vi "querey source settings menu.vi"(0 "Enable":bool=TRUE, 1 "subvi?":bool, 5 "error in (no error)":errorcluster) -> (14 "Output cluster":T2={"Integer Timestamp"=0, "Einzel Voltage"=0.0, "Needle Voltage"=0.0, "Frequency"=1.0, "Width (ms) : 0.1 "=0.05, "Desired Amplitude (V)"=0.0, "X Voltage"=0.0, "Y Voltage"=0.0, "Settings ID"="", "ID#"=0} {"Needle Voltage" min=0.0 max=10.0 step=0.01 format="%.2g"; "Y Voltage" min=0.0 max=9.0 step=0.01 format="%.2g"; "X Voltage" min=0.0 max=9.0 step=0.01 format="%.2g"; "Einzel Voltage" min=0.0 max=10.0 step=0.01 format="%.2g"; "Desired Amplitude (V)" min=0.0 max=10.0 step=0.01 format="%5.2f"; "Width (ms) : 0.1" min=0.05 max=5.0 step=0.01 format="%6.2f"; "Frequency" min=1.0 max=100.0 step=0.01 format="%.1f"}, 15 "Cancel loading":bool caption="Cancel", 18 "OK":bool, 19 "error out":errorcluster)   [LabVIEW 2012]
doc: "Displays a standard dialog box that prompts users to enter information, such as a user name and password.\n--------------------\n\nThis Express VI is configured as follows:\n\nMessage to Display to the User:\nThe inputs are: \nNumber: Upper Timestamp Range\nNumber: Lower Timestamp Range\nNumber: Settings ID"
uses:
  dust_soruce_control.ctl
  <vilib>/addons/database/Auxilliary.llb/DB Tools Cursor Type.ctl
  <vilib>/addons/database/Connection.llb/Conn Execute.vi
  <vilib>/addons/database/Recordset.llb/Rec Fetch Recordset Data (R).vi
  <vilib>/addons/database/Recordset.llb/Rec Destroy - Connection.vi
  <vilib>/addons/database/_DB Variant To Data/Database Variant To Data.xnode
  <vilib>/addons/database/NI_Database_API.lvlib
panel:
  in  "Clear Filter":bool
  in  "Tag Filter":T1
  in  "Settings ID Type":enum32{"All", "Saved", "Automatic"}(radio)
  in  "OK2":bool
  in  "Cancel":bool
  in  "Settings ID":i32(ring) items=["Any Settings ID."=-1, "Automatic Update (DT: Graphite-2-1; HV: 0.0; Time: 2/13/2014 10:09:24 AM)"=114, "Automatic Update (DT: Graphite-2-1; HV: 0.0; Time: 2/13/2014 10:09:22 AM)"=113, "Automatic Update (DT: Graphite-2-1; HV: 0.0; Time: 2/13/2014 10:09:19 AM)"=112, "Automatic Update (DT: Graphite-2-1; HV: 0.0; Time: 2/13/2014 9:57:29 AM)"=111, "Automatic Update (DT: Graphite-2-1; HV: 0.0; Time: 2/13/2014 9:57:27 AM)"=110, "Automatic Update (DT: Graphite-2-1; HV: 0.0; Time: 2/12/2014 2:14:33 PM)"=109, "Automatic Update (DT: Graphite-2-1; HV: 0.0; Time: 2/12/2014 2:14:18 PM)"=108, "Automatic Update (DT: Graphite-2-1; HV: 0.0; Time: 2/12/2014 1:53:33 PM)"=107, "Automatic Update (DT: DT: Graphite-2-1; HV: 0.0; Time: 2/12/2014 1:52:08 PM)"=106, "Automatic Update at  10/25/2012 3:24:21 PM"=100, "Automatic Update at  10/25/2012 3:14:43 PM"=99, "Automatic Update at  10/24/2012 5:17:54 PM"=98, "Automatic Update at  10/24/2012 5:05:57 PM"=96, "Automatic Update at  10/24/2012 4:27:19 PM"=95, "Automatic Update at  10/24/2012 4:13:56 PM"=94, "Automatic Update at  10/24/2012 3:47:44 PM"=90]
  in  "Lower Timestamp Range":timestamp
  in  "Upper Timestamp Range":timestamp
  out "Settings":cluster{"String":string, "Value":dbl}[](array[cluster])
  in  "Einzel Voltage":dbl
  in  "Needle Voltage":dbl
  in  "Frequency":dbl
  in  "Width (ms) : 0.1":dbl
  in  "Desired Amplitude (V)":dbl
  in  "X Voltage":dbl
  in  "Y Voltage":dbl
  out "Settings to be loaded":string
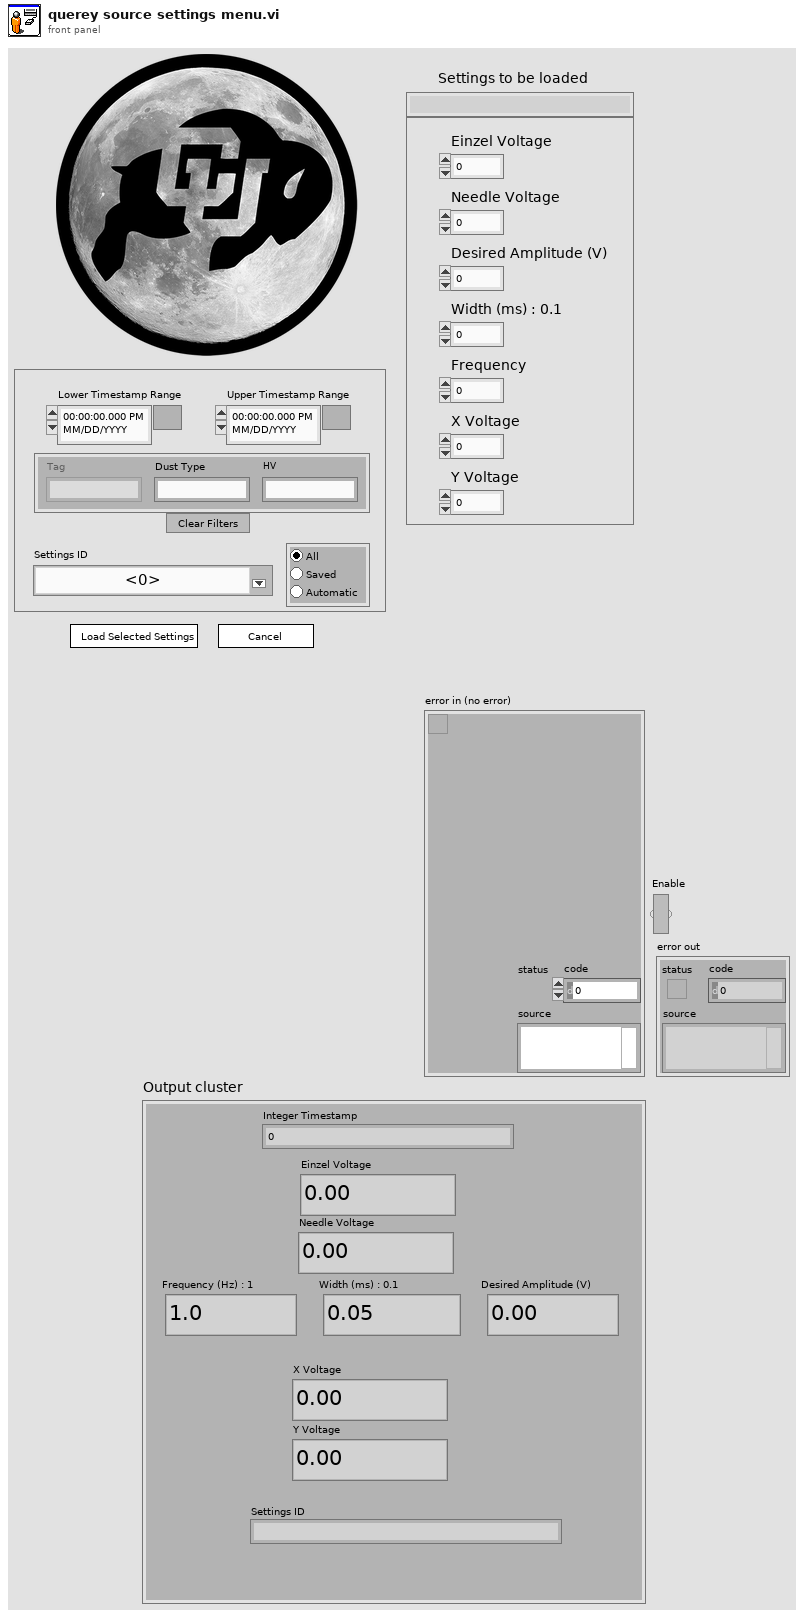
[diagram p1: front panel]
types:
  T1 = cluster{"Tag":string, "Dust Type":string, "HV":string}
  T2 = typedef "dust_soruce_control.ctl" = cluster{"Integer Timestamp":u64, "Einzel Voltage":dbl, "Needle Voltage":dbl, "Frequency":dbl, "Width (ms) : 0.1 ":dbl, "Desired Amplitude (V)":dbl, "X Voltage":dbl, "Y Voltage":dbl, "Settings ID":string, "ID#":i32}
  T3 = enum32{"Invalid", "Standard", "Closed", "Hidden", "Minimized", "Maximized"}
  T4 = enum8{"Enabled", "Disabled", "Disabled and Grayed Out"}
  T5 = typedef "NI_Database_API.lvlib/DB Tools Cursor Type.ctl" = enum16{"forward-only", "keyset", "dynamic", "static"}
  T6 = typedef "NI_Database_API.lvlib/Conn ObjectReference.ctl" = refnum<k1>
  T7 = typedef "NI_Database_API.lvlib/Rec ObjectReference.ctl" = refnum<k1>
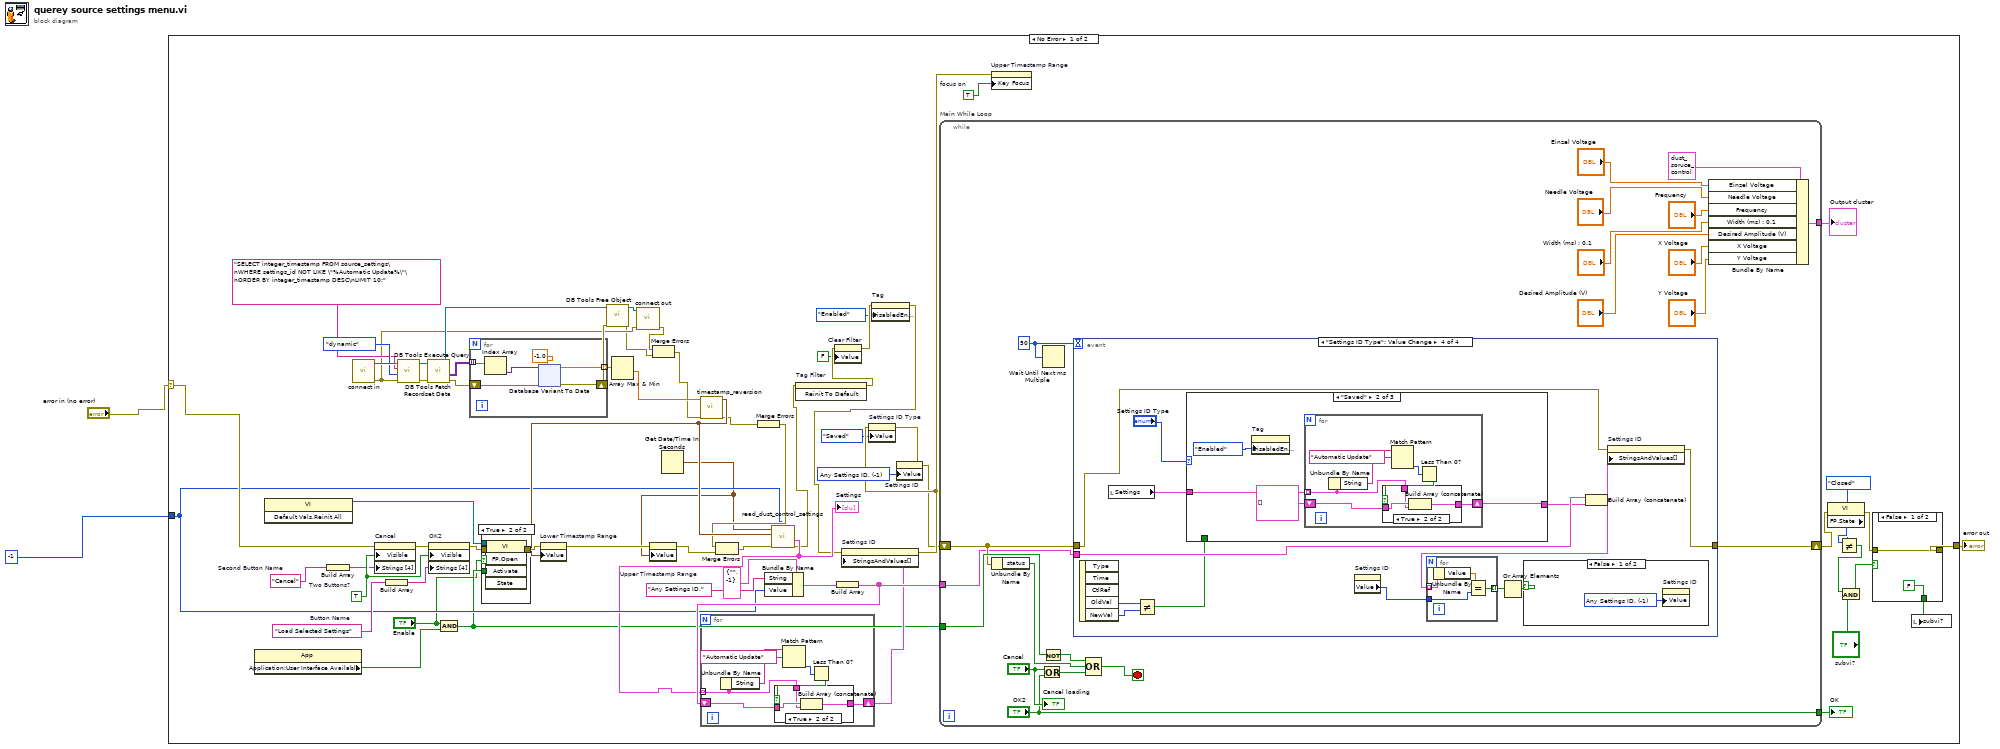
[diagram p0: block diagram]
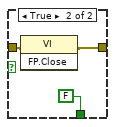
[diagram p3: hidden frame]
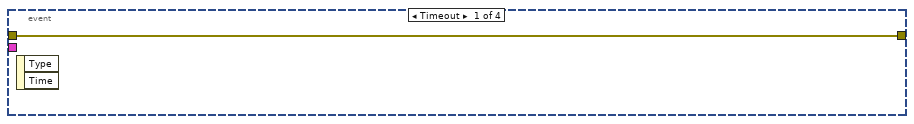
[diagram p5: hidden frame]
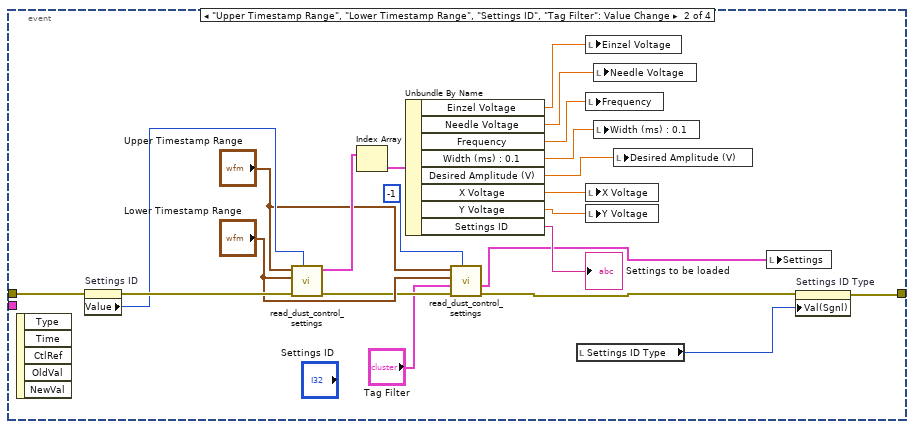
[diagram p6: hidden frame]
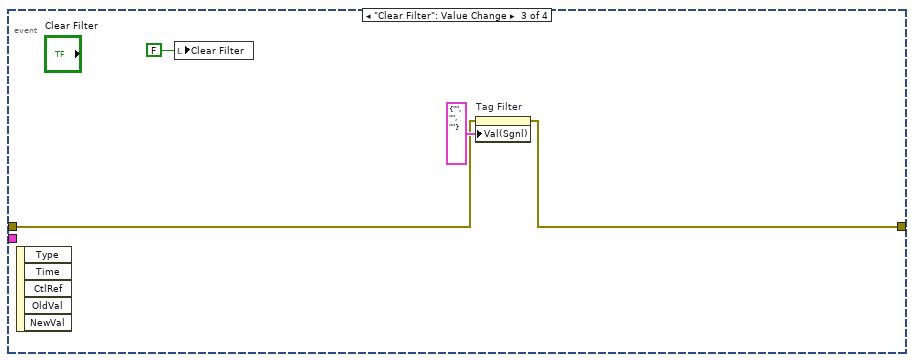
[diagram p7: hidden frame]
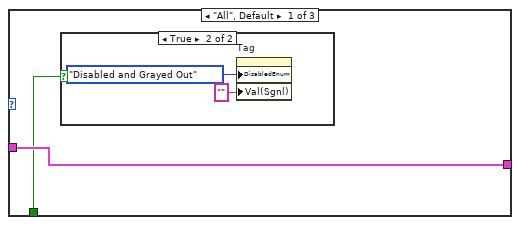
[diagram p9: hidden frame]
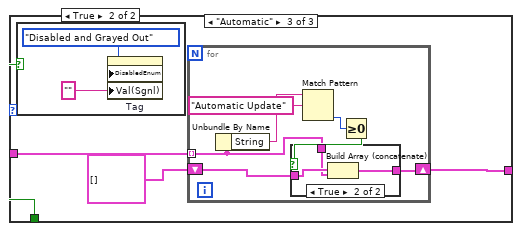
[diagram p12: hidden frame]
diagram:
  n1 = case shown="No Error" "error in (no error)" {
    selector: "error in (no error)" -> [w53 w230]
    tunnel: [w28 w230] -> w3
    tunnel: -1 ("Settings to be loaded") -> [w27 _]
    frame No Error {
      w22 = -1 items=["Any Settings ID."=-1, "Anna's Settings"=86, "Anna's Settings1"=87, "Test 'Test' \"Test\" test test."=97, "Test\""=91, "Test\""=92, "test 3"=82, "test 4"=83, "test mctesty"=88, "test mctesty"=89, "this is a \"test\" setting"=93] ("Settings ID")
      w61 = TRUE  # focus on
      w65 = "Cancel"  # Second Button Name
      w63 = "Load Selected Settings"  # Button Name
      w69 = TRUE  # Two Buttons?
      n2 = property class="App"() -> ("Application:User Interface Available"=w62:bool)  [unwired: 2 in, 2 out]
      n3 = invoke class="VI" method="Default Vals.Reinit All"() -> (reference out=w9:refnum<vi>)  [unwired: 3 in, 2 out]
      n4 = Build Array(w65) -> (w66:string[])
      n5 = call "connect in.vi"() -> ("error out"=w38:errorcluster, "Database Connection"=w48:T6)  [unwired: 7 in, 1 out]
      n6 = property on="Cancel" class="Bool"(error in=w53, "Visible"=w69, "Strings [4]"=w66) -> (error out=w67:errorcluster)  [unwired: 1 in, 1 out]
      n7 = Build Array(w63) -> (w64:string[])
      n8 = call-poly <vilib>:"DB Tools Execute Query.vi"("error in (no error)"=w38, "cursor type"=DB_Tools_Cursor_Type."dynamic", "SQL query"="SELECT integer_timestamp FROM source_settings\nWHERE settings_id NOT LIKE \"%Automatic Update%\"\nORDER BY integer_timestamp DESC\nLIMIT 10;" ("string"), "connection reference"=w48) -> ("error out"=w49:errorcluster, "recordset reference"=w50:T7)  [unwired: 4 in]
      n9 = call-poly <vilib>:"DB Tools Fetch Recordset Data.vi"("error in (no error)"=w49, "recordset reference"=w50) -> ("error out"=w44:errorcluster, "recordset data"=w45:variant[][], "recordset reference out"=w40:T7)  [unwired: 3 in]
      n10 = property on="OK2" class="Bool"(error in=w67, "Visible"=w69, "Strings [4]"=w64) -> (error out=w60:errorcluster)  [unwired: 1 in, 1 out]
      n11 = And(x="Enable", y=w62) -> (x .and. y?=w21:bool)
      n12 = for {
        tunnel: w45 -> [w95] mode=indexing
        tunnel: [w93] -> w43 mode=indexing
        shift-right: [w91] -> w39
        shift-left: w44 -> [w92]
        n13 = Index Array(array=w95) -> (element=w94:variant)  [unwired: 1 in]
        n14 = xnode "Database Variant To Data"("database variant"=w94, "error in (no error)"=w92, "type"=-1.0 ("Settings to be loaded")) -> ("data"=w93:dbl, "error out"=w91:errorcluster)
      }
      n15 = case shown="True" "Enable" {
        tunnel: w9 -> [_ w74]
        tunnel: w60 -> [w70 w73]
        tunnel: [w70 w72] -> w57
        tunnel: w21 -> [_ w71]
        frame False {
        }
        frame True {
          n16 = invoke class="VI" method="FP.Open"(reference=w74, error in=w73, "Activate"=w71) -> (error out=w72:errorcluster)  [unwired: 2 in, 4 out]
        }
      }
      n17 = call-poly <vilib>:"DB Tools Free Object.vi"("error in (no error)"=w39, "recordset reference"=w40) -> ("error out"=w37:errorcluster, "connection reference"=w41:T6)  [unwired: 8 in]
      n18 = Array Max & Min(array=w43) -> (min value=w42:dbl)  [unwired: 3 out]
      n19 = call "connect out.vi"("error in (no error)"=w38, "connection reference"=w41) -> ("error out"=w36:errorcluster)  [unwired: 9 in]
      n20 = Merge Errors(w36, w37) -> (w35:errorcluster)
      n21 = Get Date/Time In Seconds() -> (seconds since 1Jan1904=w18:timestamp)
      n22 = call "timestamp_reversion.vi"("error in (no error)"=w35, "Integer Timestamp"=w42) -> ("error out"=w33:errorcluster, "time stamp"=w34:timestamp)  [unwired: 7 in]
      n23 = property on="Lower Timestamp Range" class="AbsTime (strict)"(error in=w57, "Value"=w34) -> (error out=w58:errorcluster)  [unwired: 1 in, 1 out]
      n24 = property on="Upper Timestamp Range" class="AbsTime (strict)"(error in=w58, "Value"=w18) -> (error out=w32:errorcluster)  [unwired: 1 in, 1 out]
      n25 = Merge Errors(w33) -> (w31:errorcluster)
      n26 = Merge Errors(w31, w32) -> (w30:errorcluster)
      n27 = Bundle By Name(cluster=cluster{"String":string, "Value":i32} {"String"="", "Value"=-1}, "String"="Any Settings ID." ("Settings to be loaded"), "Value"=w27) -> (w54:cluster{"String":string, "Value":i32})
      n28 = call "read_dust_control_settings.vi"("Settings to be loaded"=w27, "error in (no error)"=w30, "Lower Timestamp Range"=w34, "Upper Timestamp Range"=w18) -> ("error out"=w17:errorcluster, "Array"=w25:cluster{"String":string, "Value":dbl}[])  [unwired: 5 in, 1 out]
      "Settings" <- w25
      n29 = invoke on="Tag Filter" class="Clust (strict)" method="Reinit To Default"(error in=w17) -> (error out=w16:errorcluster)  [unwired: 2 in, 2 out]
      n30 = property on="Clear Filter" class="Bool (strict)"(error in=w16, "Value"=FALSE ("Clear Filter")) -> (error out=w14:errorcluster)  [unwired: 1 in, 1 out]
      n31 = Build Array(w54) -> (w29:cluster{"String":string, "Value":i32}[])
      n32 = for {
        tunnel: w25 -> [w82] mode=indexing
        shift-right: [w81] -> w26
        shift-left: w29 -> [w83]
        n33 = Unbundle By Name(w82) -> ("String"=w86:string)
        n34 = Match Pattern(string=w86, regular expression="Automatic Update") -> (offset past match=w80:i32)  [unwired: 1 in, 3 out]
        n35 = Less Than 0?(x=w80) -> (x < 0?=w84:bool)
        n36 = case shown="True" w84 {
          tunnel: w83 -> [w87 w90]
          tunnel: w82 -> [_ w89]
          tunnel: [w87 w88] -> w81
          frame False {
          }
          frame True {
            n37 = Build Array (concatenate)(w90, w89) -> (w88:cluster{"String":string, "Value":dbl}[])
          }
        }
      }
      n38 = property on="Tag" class="Str"(error in=w14, "DisabledEnum"=T4."Enabled" ("Disabled")) -> (error out=w12:errorcluster)  [unwired: 1 in, 1 out]
      n39 = property on="Settings ID" class="Ring (strict)"(error in=w12, "StringsAndValues[]"=w26) -> (error out=w52:errorcluster)  [unwired: 1 in, 1 out]
      n40 = property on="Settings ID Type" class="RadioBtnsControl (strict)"(error in=w52, "Value"=enum32{"All", "Saved", "Automatic"}."Saved" ("Settings ID Type")) -> (error out=w24:errorcluster)  [unwired: 1 in, 1 out]
      n41 = property on="Settings ID" class="Ring (strict)"(error in=w24, "Value"=w22) -> (error out=w23:errorcluster)  [unwired: 1 in, 1 out]
      n42 = while "Main While Loop" {
        tunnel: ["OK2"] -> w68
        tunnel: w21 -> [w147]
        tunnel: w29 -> [w129]
        tunnel: [w138] -> w59
        shift-right: [w140] -> w8
        shift-left: w23 -> [w141]
        stop <- w145 stop-if-true
        w139 = u32 50 ("millisecond multiple")
        n43 = Unbundle By Name(w141) -> ("status"=w143:bool)
        n44 = Or(x="Cancel", y="OK2") -> (x .or. y?=w144:bool)
        n45 = Not(x=w147) -> (.not. x?=w146:bool)
        n46 = Wait Until Next ms Multiple(millisecond multiple=w139) -> ()  [unwired: 1 out]
        n47 = event shown="[3] \"Settings ID Type\": Value Change" {
          selector: _ -> [_ _ _ _]
          dyn-events: _ -> [_ _ _ _]
          timeout: w139 -> [_ _ _ _]
          tunnel: w141 -> [w149 w171 w173 w186]
          tunnel: [w149 w152 w172 w185] -> w140
          tunnel: w129 -> [_ _ _ w180]
          event Timeout {
            n48 = event-data() -> ()  [unwired: 1 in, 2 out]
          }
          event "Upper Timestamp Range", "Lower Timestamp Range", "Settings ID", "Tag Filter": Value Change {
            n49 = event-data() -> ()  [unwired: 1 in, 5 out]
            n50 = property on="Settings ID" class="Ring (strict)"(error in=w171) -> (error out=w170:errorcluster, "Value"=w168:i32)  [unwired: 1 in, 1 out]
            n51 = call "read_dust_control_settings.vi"("Settings to be loaded"=w168, "error in (no error)"=w170, "Lower Timestamp Range"="Lower Timestamp Range", "Upper Timestamp Range"="Upper Timestamp Range") -> ("error out"=w165:errorcluster, "Dust Source Array"=w169:T2[])  [unwired: 5 in, 1 out]
            n52 = Index Array(array=w169) -> (element=w164:T2)  [unwired: 1 in]
            n53 = Unbundle By Name(w164) -> ("Einzel Voltage"=w163:dbl, "Needle Voltage"=w162:dbl, "Frequency"=w161:dbl, "Width (ms) : 0.1"=w160:dbl, "Desired Amplitude (V)"=w159:dbl, "X Voltage"=w158:dbl, "Y Voltage"=w157:dbl, "Settings ID"=→"Settings to be loaded":string)
            n54 = call "read_dust_control_settings.vi"("Settings to be loaded"=-1, "error in (no error)"=w165, "Cluster"="Tag Filter", "Lower Timestamp Range"="Lower Timestamp Range", "Upper Timestamp Range"="Upper Timestamp Range") -> ("error out"=w153:errorcluster, "Array"=w151:cluster{"String":string, "Value":dbl}[])  [unwired: 4 in, 1 out]
            n55 = local read "Settings ID Type"() -> (w154:enum32{"All", "Saved", "Automatic"})
            n56 = local write "Einzel Voltage"(w163) -> ()
            n57 = local write "Frequency"(w161) -> ()
            n58 = local write "X Voltage"(w158) -> ()
            n59 = local write "Y Voltage"(w157) -> ()
            n60 = local write "Needle Voltage"(w162) -> ()
            n61 = local write "Width (ms) : 0.1"(w160) -> ()
            n62 = local write "Desired Amplitude (V)"(w159) -> ()
            n63 = local write "Settings"(w151) -> ()
            n64 = property on="Settings ID Type" class="RadioBtnsControl (strict)"(error in=w153, "Val(Sgnl)"=w154) -> (error out=w152:errorcluster)  [unwired: 1 in, 1 out]
          }
          event "Clear Filter": Value Change {
            n65 = event-data() -> ()  [unwired: 1 in, 5 out]
            n66 = local write "Clear Filter"(FALSE ("Clear Filter")) -> ()
            n67 = property on="Tag Filter" class="Clust (strict)"(error in=w173, "Val(Sgnl)"=T1 {"Tag"="", "Dust Type"="", "HV"=""} ("Value (Signaling)")) -> (error out=w172:errorcluster)  [unwired: 1 in, 1 out]
          }
          event "Settings ID Type": Value Change {
            n68 = event-data() -> ("OldVal"=w178:enum32{"All", "Saved", "Automatic"}, "NewVal"=w177:enum32{"All", "Saved", "Automatic"})  [unwired: 1 in, 3 out]
            n69 = local read "Settings"() -> (w187:cluster{"String":string, "Value":dbl}[])
            n70 = Not Equal?(x=w178, y=w177) -> (x != y?=w176:bool)
            n71 = case shown="\"Saved\"" "Settings ID Type" {
              tunnel: w187 -> [w195 w201 w216]
              tunnel: [w195 w199 w215] -> w179
              tunnel: w176 -> [w194 _ w213]
              frame "All", Default {
                n72 = case shown="True" w194 {
                  frame False {
                  }
                  frame True {
                    n73 = property on="Tag" class="Str"("DisabledEnum"=T4."Disabled and Grayed Out" ("Disabled"), "Val(Sgnl)"="" ("Value")) -> ()  [unwired: 2 in, 2 out]
                  }
                }
              }
              frame "Saved" {
                n74 = property on="Tag" class="Str"("DisabledEnum"=T4."Enabled" ("Disabled")) -> ()  [unwired: 2 in, 2 out]
                n75 = for {
                  tunnel: w201 -> [w203] mode=indexing
                  shift-right: [w202] -> w199
                  shift-left: cluster{"String":string, "Value":i32}[] [] -> [w204]
                  n76 = Unbundle By Name(w203) -> ("String"=w208:string)
                  n77 = Match Pattern(string=w208, regular expression="Automatic Update") -> (offset past match=w206:i32)  [unwired: 1 in, 3 out]
                  n78 = Less Than 0?(x=w206) -> (x < 0?=w205:bool)
                  n79 = case shown="True" w205 {
                    tunnel: w204 -> [w209 w212]
                    tunnel: w203 -> [_ w211]
                    tunnel: [w209 w210] -> w202
                    frame False {
                    }
                    frame True {
                      n80 = Build Array (concatenate)(w212, w211) -> (w210:cluster{"String":string, "Value":dbl}[])
                    }
                  }
                }
              }
              frame "Automatic" {
                n81 = case shown="True" w213 {
                  frame False {
                  }
                  frame True {
                    n82 = property on="Tag" class="Str"("DisabledEnum"=T4."Disabled and Grayed Out" ("Disabled"), "Val(Sgnl)"="" ("Value")) -> ()  [unwired: 2 in, 2 out]
                  }
                }
                n83 = for {
                  tunnel: w216 -> [w220] mode=indexing
                  shift-right: [w219] -> w215
                  shift-left: cluster{"String":string, "Value":i32}[] [] -> [w221]
                  n84 = Unbundle By Name(w220) -> ("String"=w225:string)
                  n85 = Match Pattern(string=w225, regular expression="Automatic Update") -> (offset past match=w223:i32)  [unwired: 1 in, 3 out]
                  n86 = Greater Or Equal To 0?(x=w223) -> (x >= 0?=w222:bool)
                  n87 = case shown="True" w222 {
                    tunnel: w221 -> [w226 w229]
                    tunnel: w220 -> [_ w228]
                    tunnel: [w226 w227] -> w219
                    frame False {
                    }
                    frame True {
                      n88 = Build Array (concatenate)(w229, w228) -> (w227:cluster{"String":string, "Value":dbl}[])
                    }
                  }
                }
              }
            }
            n89 = property on="Settings ID" class="Ring (strict)"() -> ("Value"=w184:i32)  [unwired: 2 in, 2 out]
            n90 = Build Array (concatenate)(w180, w179) -> (w181:cluster{"String":string, "Value":dbl}[])
            n91 = for {
              tunnel: w181 -> [w192] mode=indexing
              tunnel: w184 -> [w190]
              tunnel: [w189] -> w183 mode=indexing
              n92 = Unbundle By Name(w192) -> ("Value"=w191:dbl)
              n93 = Equal?(x=w191, y=w190) -> (x = y?=w189:bool)
            }
            n94 = Or Array Elements(Boolean array=w183) -> (logical OR=w182:bool)
            n95 = case shown="False" w182 {
              frame False {
                w193 = i16 -1 items=["Any Settings ID."=-1, "Anna's Settings"=86, "Anna's Settings1"=87, "Test 'Test' \"Test\" test test."=97, "Test\""=91, "Test\""=92, "test 3"=82, "test 4"=83, "test mctesty"=88, "test mctesty"=89, "this is a \"test\" setting"=93] ("Settings ID")
                n96 = property on="Settings ID" class="Ring (strict)"("Value"=w193) -> ()  [unwired: 2 in, 2 out]
              }
              frame True {
              }
            }
            n97 = property on="Settings ID" class="Ring (strict)"(error in=w186, "StringsAndValues[]"=w181) -> (error out=w185:errorcluster)  [unwired: 1 in, 1 out]
          }
        }
        n98 = Compound Arithmetic op=OR(w146, w143, w144) -> (w145:bool)
        n99 = Bundle By Name(cluster=T2 {"Integer Timestamp"=0, "Einzel Voltage"=0.0, "Needle Voltage"=0.0, "Frequency"=1.0, "Width (ms) : 0.1 "=0.05, "Desired Amplitude (V)"=0.0, "X Voltage"=0.0, "Y Voltage"=0.0, "Settings ID"="", "ID#"=0} ("Output cluster"), "Einzel Voltage"="Einzel Voltage", "Needle Voltage"="Needle Voltage", "Frequency"="Frequency", "Width (ms) : 0.1"="Width (ms) : 0.1", "Desired Amplitude (V)"="Desired Amplitude (V)", "X Voltage"="X Voltage", "Y Voltage"="Y Voltage") -> (w138:T2)
        "Cancel loading" <- "Cancel"
      }
      "OK" <- w68
      "Output cluster" <- w59
      n100 = property on="Upper Timestamp Range" class="AbsTime (strict)"(error in=w52, "Key Focus"=w61) -> ()  [unwired: 1 in, 2 out]
      n101 = property class="VI"(error in=w8) -> (error out=w7:errorcluster, "FP.State"=w6:T3)  [unwired: 1 in, 1 out]
      n102 = Not Equal?(x=w6, y=T3."Closed") -> (x != y?=w4:bool)
      n103 = And(x=w4, y="subvi?") -> (x .and. y?=w10:bool)
      n104 = case shown="False" w10 {
        tunnel: w7 -> [w76 w79]
        tunnel: [w76 w78] -> w28
        tunnel: [FALSE ("subvi?") FALSE ("subvi?")] -> w11
        frame False {
        }
        frame True {
          n105 = invoke class="VI" method="FP.Close"(error in=w79) -> (error out=w78:errorcluster)  [unwired: 2 in, 2 out]
        }
      }
      n106 = local write "subvi?"(w11) -> ()
    }
    frame Error {
    }
  }
  "error out" <- w3
